vi "_062.vi"() -> ()   [LabVIEW 2024]
uses:
  <vilib>/Utility/file.llb/Write Delimited Spreadsheet (string).vi
panel:
  out "transposed array":string[][](array[string])
  in  "file path (dialog if empty)":path
  in  "Array 3":string[](array[string])
  out "F-format string":string[][](array[string])
  in  "Array 2":string[](array[string])
  out "Array":dbl[][](array[numeric])
  # "To Bring the data in correct manner :"
  # "( Data Acquisition )"
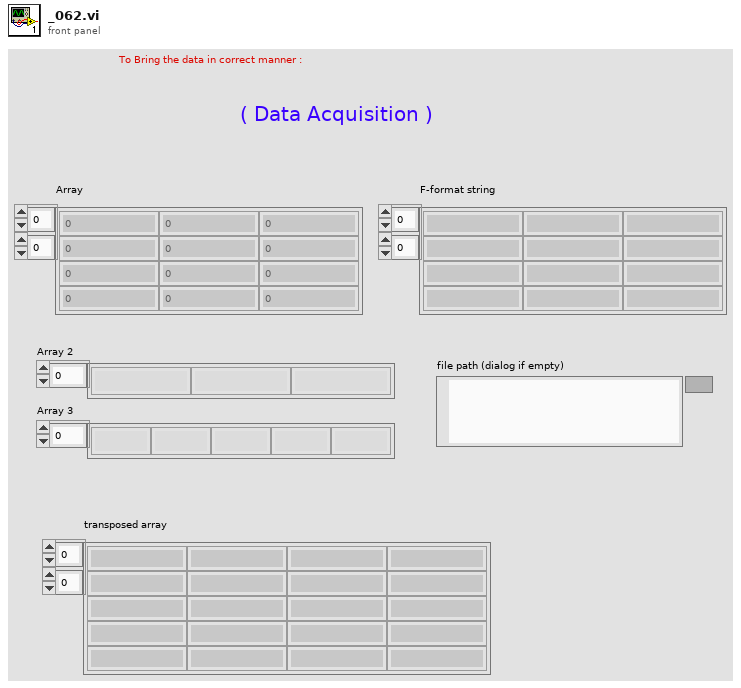
[diagram p1: front panel]
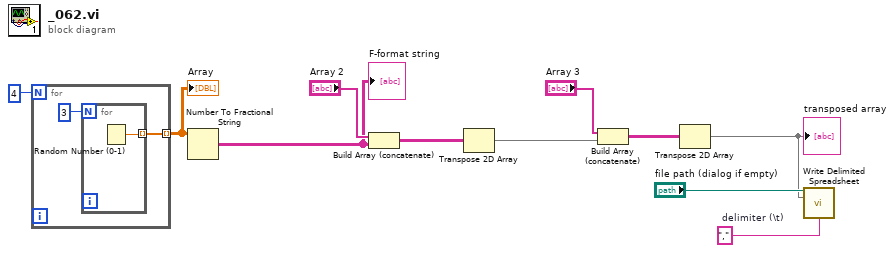
[diagram p0: block diagram]
diagram:
  w2 = ","  # delimiter (\t)
  n1 = for {
    N: 4 -> [_]
    tunnel: [w12] -> w10 mode=indexing
    n2 = for {
      N: 3 -> [_]
      tunnel: [w14] -> w12 mode=indexing
      n3 = Random Number (0-1)() -> (number: 0 to 1=w14:dbl)
    }
  }
  "Array" <- w10
  n4 = Number To Fractional String(number=w10) -> (F-format string=w7:string[][])  [unwired: 3 in]
  "F-format string" <- w7
  n5 = Build Array (concatenate) "Build Array"("Array 2", w7) -> (w5:string[][])
  n6 = Transpose 2D Array(2D array=w5) -> (transposed array=w4:string[][])
  n7 = Build Array (concatenate) "Build Array"("Array 3", w4) -> (w3:string[][])
  n8 = Transpose 2D Array(2D array=w3) -> (transposed array=w1:string[][])
  "transposed array" <- w1
  n9 = call-poly <vilib>:"Write Delimited Spreadsheet.vi"("file path (dialog if empty)"="file path (dialog if empty)", "2D data"=w1, "delimiter (\\t)"=w2) -> ()  [unwired: 11 in, 2 out]
